vi "_caraya_renameOperands.vi"(8 "error in (no error)":errorcluster, 10 "Application":refnum<vi>, 11 "New Class Path":path=path "C:/Projects/JKI/Caraya/src/tests/test-all-asserts/Test Runner.AllAsserts.lvclass") -> (0 "error out":errorcluster)   [LabVIEW 2013]
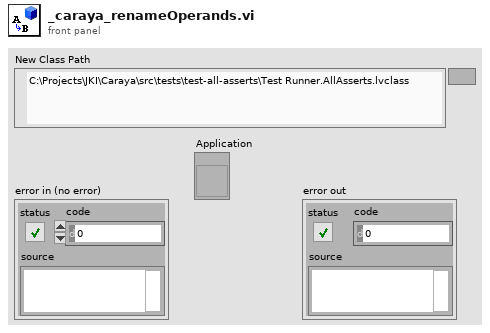
[diagram p1: front panel]
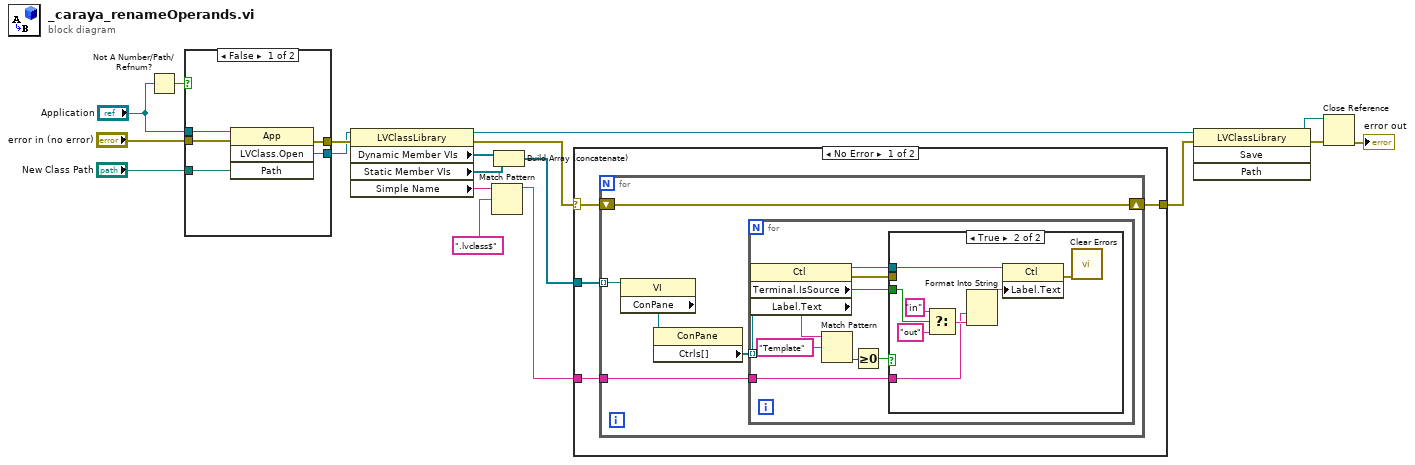
[diagram p0: block diagram]
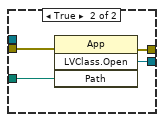
[diagram p4: hidden frame]
diagram:
  n1 = Not A Number/Path/Refnum?(number/path/refnum="Application") -> (NaN/Path/Refnum?=w6:bool)
  n2 = case shown="False" w6 {
    tunnel: [w23 w27] -> w14
    tunnel: [w22 w26] -> w12
    tunnel: "New Class Path" -> [w21 w25]
    tunnel: "error in (no error)" -> [w20 w24]
    tunnel: "Application" -> [w19 _]
    frame False {
      n3 = invoke class="App" method="LVClass.Open"(reference=w19, error in=w20, "Path"=w21) -> (error out=w23:errorcluster, "LVClass.Open"=w22:refnum<vi>)  [unwired: 1 in, 2 out]
    }
    frame True {
      n4 = invoke class="App" method="LVClass.Open"(error in=w24, "Path"=w25) -> (error out=w27:errorcluster, "LVClass.Open"=w26:refnum<vi>)  [unwired: 2 in, 2 out]
    }
  }
  n5 = property class="LVClassLibrary"(reference=w12, error in=w14) -> (reference out=w13:refnum<vi>, error out=w2:errorcluster, "Dynamic Member VIs"=w18:refnum<vi>[], "Static Member VIs"=w17:refnum<vi>[], "Simple Name"=w4:string)
  n6 = Match Pattern(string=w4, regular expression=".lvclass$") -> (before substring=w3:string)  [unwired: 1 in, 3 out]
  n7 = Build Array (concatenate)(w18, w17) -> (w16:refnum<vi>[])
  n8 = case shown="No Error" w2 {
    selector: w2 -> [w28 w54]
    tunnel: w16 -> [w31 _]
    tunnel: [w30 w54] -> w10
    tunnel: w3 -> [w29 _]
    frame No Error {
      n9 = for {
        tunnel: w31 -> [w36] mode=indexing
        shift-right: [w33] -> w30
        shift-left: w28 -> [w33]
        tunnel: w29 -> [w32]
        n10 = property class="VI"(reference=w36) -> ("ConPane"=w35:refnum<vi>)  [unwired: 1 in, 2 out]
        n11 = property class="ConPane"(reference=w35) -> ("Ctrls[]"=w34:refnum<vi>[])  [unwired: 1 in, 2 out]
        n12 = for {
          tunnel: w34 -> [w45] mode=indexing
          tunnel: w32 -> [w38]
          n13 = property class="Ctl"(reference=w45) -> (reference out=w39:refnum<vi>, error out=w37:errorcluster, "Terminal.IsSource"=w40:bool, "Label.Text"=w44:string)  [unwired: 1 in]
          n14 = Match Pattern(string=w44, regular expression="Template") -> (offset past match=w42:i32)  [unwired: 1 in, 3 out]
          n15 = Greater Or Equal To 0?(x=w42) -> (x >= 0?=w41:bool)
          n16 = case shown="True" w41 {
            tunnel: w40 -> [_ w51]
            tunnel: w39 -> [_ w50]
            tunnel: w38 -> [_ w47]
            tunnel: w37 -> [_ _]
            frame False {
            }
            frame True {
              n17 = Select(t="in" ("regular expression"), s=w51, f="out" ("regular expression")) -> (s? t:f=w48:string)
              n18 = Format Into String(w47, w48) -> (resulting string=w46:string)  [unwired: 3 in, 1 out]
              n19 = property class="Ctl"(reference=w50, "Label.Text"=w46) -> (error out=w49:errorcluster)  [unwired: 1 in, 1 out]
              n20 = call <vilib>:"Clear Errors.vi"("error in (no error)"=w49) -> ()  [unwired: 6 in, 1 out]
            }
          }
        }
      }
    }
    frame Error {
    }
  }
  n21 = invoke class="LVClassLibrary" method="Save"(reference=w13, error in=w10) -> (reference out=w1:refnum<vi>, error out=w15:errorcluster)  [unwired: 2 in, 2 out]
  n22 = Close Reference(reference=w1, error in (no error)=w15) -> (error out=→"error out":errorcluster)
